vi "Read Data.vi"(8 "error in (no error)":errorcluster, 11 "EK-P4 in":refnum<class "EK-P4.lvclass">) -> (0 "error out":errorcluster, 1 "NumberOfMeasuredPackagesLost":u32, 2 "Data":dbl[](array[numeric]), 3 "EK-P4 out":refnum<class "EK-P4.lvclass">, 5 "NumberOfMeasurements":u16)   [LabVIEW 2016, in "EK-P4.lvclass"]
doc: "read continuous data from the EK-P4 board. Needs to be called in a while loop."
uses:
  EK-P4.lvclass
  UsbScShdlc_Sensirion/control/InterlacedDataSF06_UsbScShdlc_Sensirion.ctl
  EK-P4.lvclass/EK-P4.ctl
  <vilib>/Utility/error.llb/Error Cluster From Error Code.vi
  <vilib>/ErrorRing/Error Ring.xnode
panel:
  out "InterlacedDataSF06":T1
  out "NumberOfPackagesRemainingInBuffer":u16
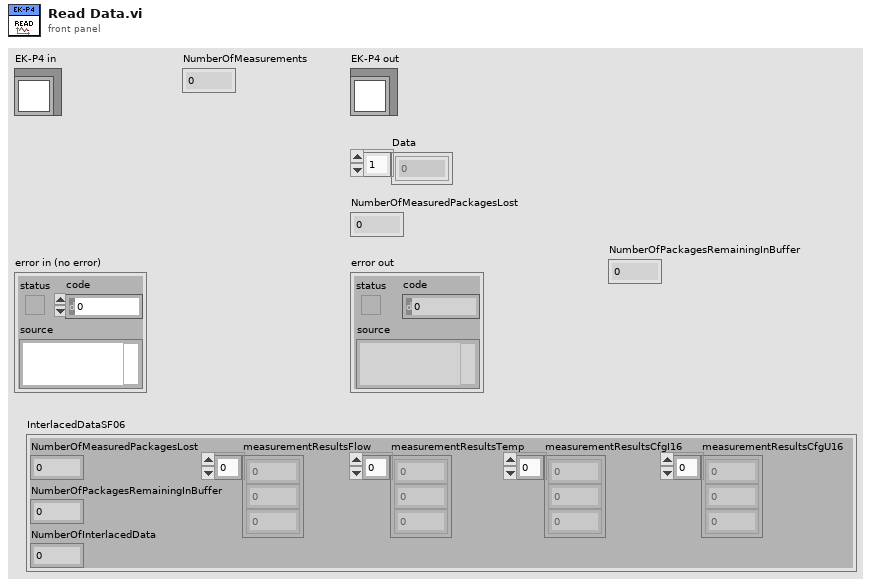
[diagram p1: front panel]
types:
  T1 = typedef "InterlacedDataSF06_UsbScShdlc_Sensirion.ctl" = cluster{"NumberOfMeasuredPackagesLost":u32, "NumberOfPackagesRemainingInBuffer":u16, "NumberOfInterlacedData":u16, "measurementResultsFlow":i16[], "measurementResultsTemp":i16[], "measurementResultsCfgI16":i16[], "measurementResultsCfgU16":u16[]}
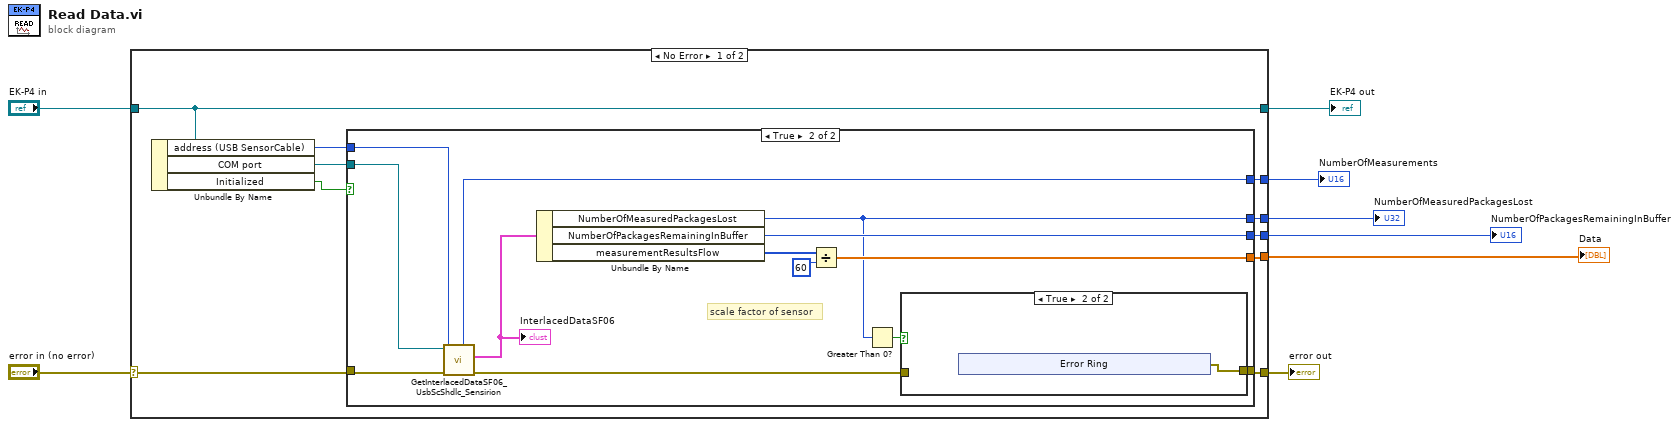
[diagram p0: block diagram]
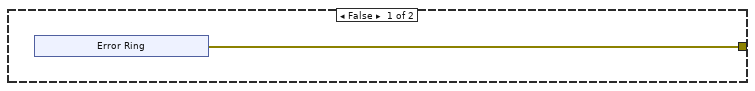
[diagram p2: hidden frame]
diagram:
  n1 = case shown="No Error" "error in (no error)" {
    selector: "error in (no error)" -> [w18 w46]
    tunnel: [w17 w46] -> w7
    tunnel: [w16 w45] -> w5
    tunnel: "EK-P4 in" -> [w16 w45]
    tunnel: [w13 _] -> w4
    tunnel: [w12 _] -> w3
    tunnel: [w11 _] -> w2
    tunnel: [w10 _] -> w1
    frame No Error {
      n2 = Unbundle By Name(w16) -> ("address (USB SensorCable)"=w14:u8, "COM port"=w15:refnum<visa-resource-name>, "Initialized"=w9:bool)
      n3 = case shown="True" w9 {
        tunnel: w18 -> [_ w37]
        tunnel: [w19 w27] -> w17
        tunnel: w15 -> [_ w36]
        tunnel: w14 -> [_ w35]
        tunnel: [_ w33] -> w13
        tunnel: [_ w25] -> w12
        tunnel: [_ w32] -> w11
        tunnel: [_ w29] -> w10
        frame False {
          n4 = xnode "Error Ring"() -> ("error out"=w19:errorcluster)
        }
        frame True {
          # "scale factor of sensor"
          n5 = call "GetInterlacedDataSF06_UsbScShdlc_Sensirion.vi"("address"=w35, "error in (no error)"=w37, "COM port"=w36) -> ("error out"=w28:errorcluster, "InterlacedDataSF06"=w34:T1, "ReadDataSets"=w33:u16)  [unwired: 5 in, 1 out]
          "InterlacedDataSF06" <- w34
          n6 = Unbundle By Name(w34) -> ("NumberOfMeasuredPackagesLost"=w25:u32, "NumberOfPackagesRemainingInBuffer"=w32:u16, "measurementResultsFlow"=w30:i16[])
          n7 = Divide(x=w30, y=u16 60 ("ScaleFactor flow/dp")) -> (x/y=w29:dbl[])
          n8 = Greater Than 0?(x=w25) -> (x > 0?=w26:bool)
          n9 = case shown="True" w26 {
            tunnel: w28 -> [w38 _]
            tunnel: [w38 w39] -> w27
            frame False {
            }
            frame True {
              n10 = xnode "Error Ring"() -> ("error out"=w39:errorcluster)
            }
          }
        }
      }
    }
    frame Error {
    }
  }
  "error out" <- w7
  "EK-P4 out" <- w5
  "NumberOfMeasurements" <- w4
  "NumberOfMeasuredPackagesLost" <- w3
  "NumberOfPackagesRemainingInBuffer" <- w2
  "Data" <- w1
